vi "SetFreqOffset.vi"(6 "Resp Timeout (ms)":i32 min=0, 7 "Enum":T1, 8 "Error In":errorcluster, 10 "Freq Offset (Hz)":i64=1, 11 "FPGA Reference":refnum<k20>) -> (0 "Error Out":errorcluster, 1 "Received Text":string, 2 "Set Freq Offset OK":bool)   [LabVIEW 2018]
uses:
  Resources_Test/UART/ControlTestSlot.ctl
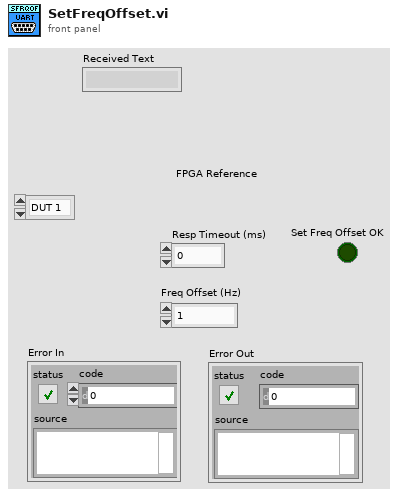
[diagram p1: front panel]
types:
  T1 = typedef "ControlTestSlot.ctl" = enum16{"DUT 1", "DUT 2"}
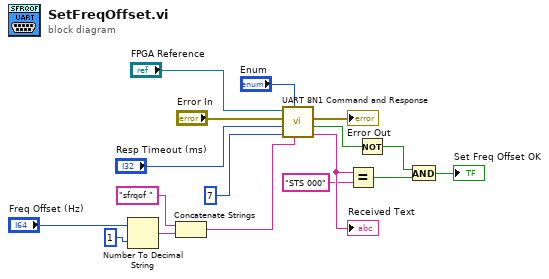
[diagram p0: block diagram]
diagram:
  n1 = Number To Decimal String(number="Freq Offset (Hz)", width (-)=i16 1) -> (decimal integer string=w11:string)
  n2 = Concatenate Strings("sfrqof " ("Text to Send"), w11) -> (w5:string)
  n3 = call "UART 8N1 Command and Response.vi"("Text to Send"=w5, "Active Dut"="Enum", "Response Size (char)"=u32 7, "Response Timeout (ms)"="Resp Timeout (ms)", "Error In"="Error In", "FPGA VI Reference In"="FPGA Reference") -> ("Received Text"=w2:string, "Timeout Flag"=w3:bool, "Error Out"=→"Error Out":errorcluster)  [unwired: 2 in, 1 out]
  "Received Text" <- w2
  n4 = Equal?(x=w2, y="STS 000") -> (x = y?=w15:bool)
  n5 = Not(x=w3) -> (.not. x?=w17:bool)
  n6 = And(x=w17, y=w15) -> (x .and. y?=→"Set Freq Offset OK":bool)
